vi "Report Shake Data.vi"(8 "error in (no error)":errorcluster, 9 "Amplitude (g)":dbl, 10 "Frequency (Hz)":dbl, 11 "Shaker Controller Interface in":refnum<class "Shaker Controller Interface.lvclass">) -> (0 "error out":errorcluster, 3 "Shaker Controller Interface out":refnum<class "Shaker Controller Interface.lvclass">)   [LabVIEW 2020, in "Shaker Controller Interface.lvlib" / "Shaker Controller Interface.lvclass"]
uses:
  Shaker Controller Interface.lvclass
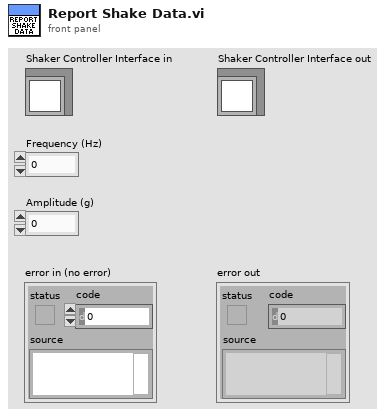
[diagram p1: front panel]
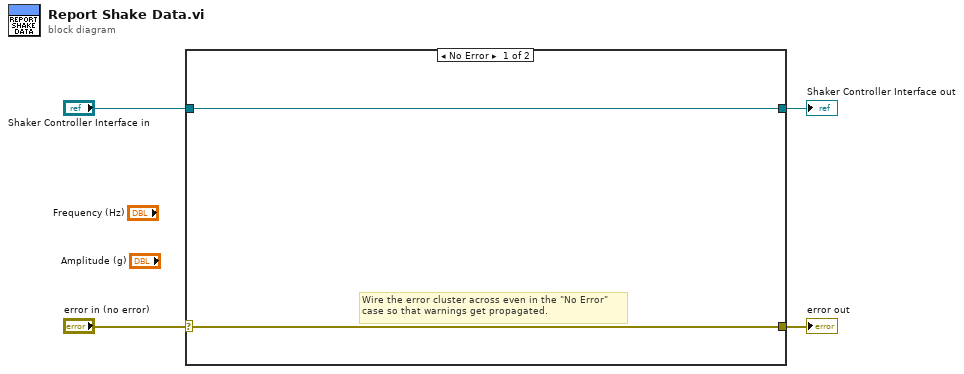
[diagram p0: block diagram]
diagram:
  n1 = case shown="No Error" "error in (no error)" {
    selector: "error in (no error)" -> [w5 w8]
    tunnel: [w5 w8] -> w3
    tunnel: [w6 w7] -> w1
    tunnel: "Shaker Controller Interface in" -> [w6 w7]
    frame No Error {
      # "Wire the error cluster across even in the \"No Error\"\ncase so that warnings get propagated."
    }
    frame Error {
    }
  }
  "error out" <- w3
  "Shaker Controller Interface out" <- w1
